vi "Get Width.vi"(8 "Error In":errorcluster, 11 "Square In":refnum<class "Square.lvclass">) -> (0 "Error Out":errorcluster, 2 "Width":u32, 3 "Square Out":refnum<class "Square.lvclass">)   [LabVIEW 2019, in "Square.lvclass"]
uses:
  Square.lvclass
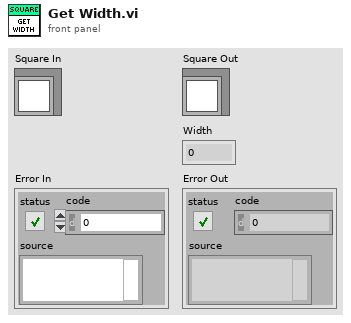
[diagram p1: front panel]
types:
  T1 = typedef "Square.lvclass/Data.ctl" = cluster{"Height":u32, "Width":u32}
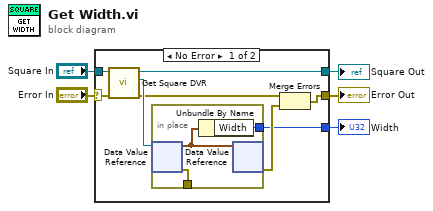
[diagram p0: block diagram]
diagram:
  n1 = case shown="No Error" "Error In" {
    selector: "Error In" -> [w9 w17]
    tunnel: [w11 w17] -> w4
    tunnel: [w7 w18] -> w2
    tunnel: "Square In" -> [w10 w18]
    tunnel: [w12 _] -> w1
    frame No Error {
      n2 = call "Get Square DVR.vi"("Error In"=w9, "Square In"=w10) -> ("Error Out"=w6:errorcluster, "DVR"=w8:refnum<data-value>, "Square Out"=w7:refnum<class "Square.lvclass">)  [unwired: 7 in]
      n3 = in-place {
        in-place-border: [w14] -> w12
        in-place-border: [w16] -> _
        n4 = in-place-dvr #1(w8) -> (w15:T1, w16:errorcluster)
        n5 = Unbundle By Name(w15) -> ("Width"=w14:u32)
        n6 = in-place-dvr #1(w15) -> (w13:errorcluster)  [unwired: 1 out]
      }
      n7 = Merge Errors(w6, w13) -> (w11:errorcluster)
    }
    frame Error {
    }
  }
  "Square Out" <- w2
  "Error Out" <- w4
  "Width" <- w1
